vi "XVC_SERVER_UDPV3.vi"() -> ()   [LabVIEW 2017]
panel:
  out "字符串 3":string
  out "错误输出 3":errorcluster={"status"=TRUE, "code"=56, "source"="XVC_SERVER_UDPV3.vi中的读取TCP数据"} caption="错误输出"
  out "错误输出":errorcluster
  in  "address":string="192.168.10.35"
  out "x != 0?":bool=TRUE
  in  "Client Closed":string="The client VI closed the connection."
  in  "Stop":bool
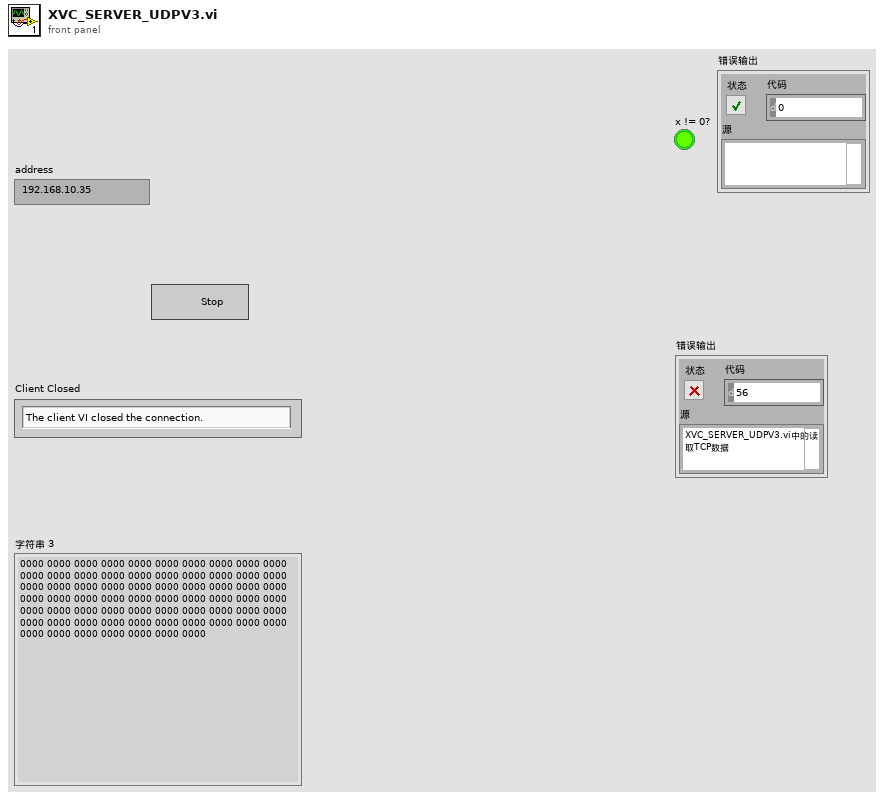
[diagram p1: front panel]
types:
  T1 = enum16{"Standard", "Buffered", "CRLF", "Immediate"}
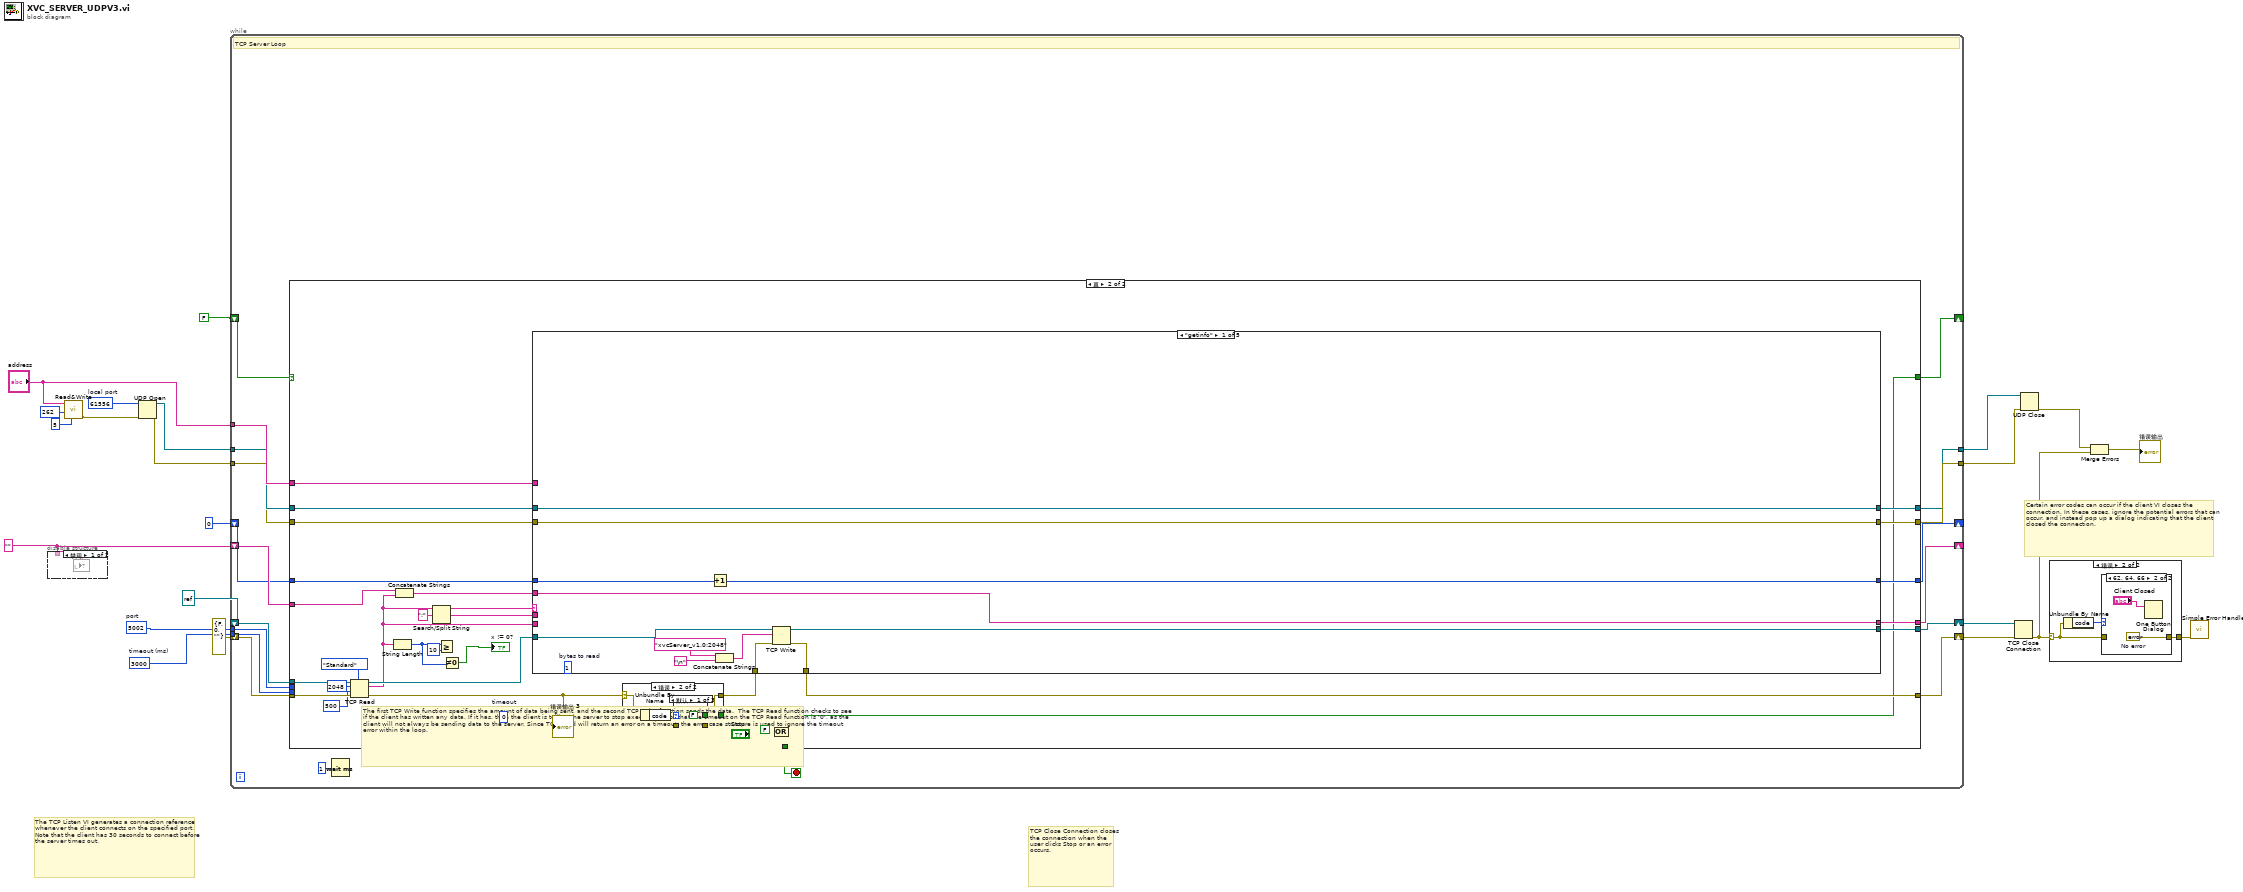
[diagram p0: block diagram]
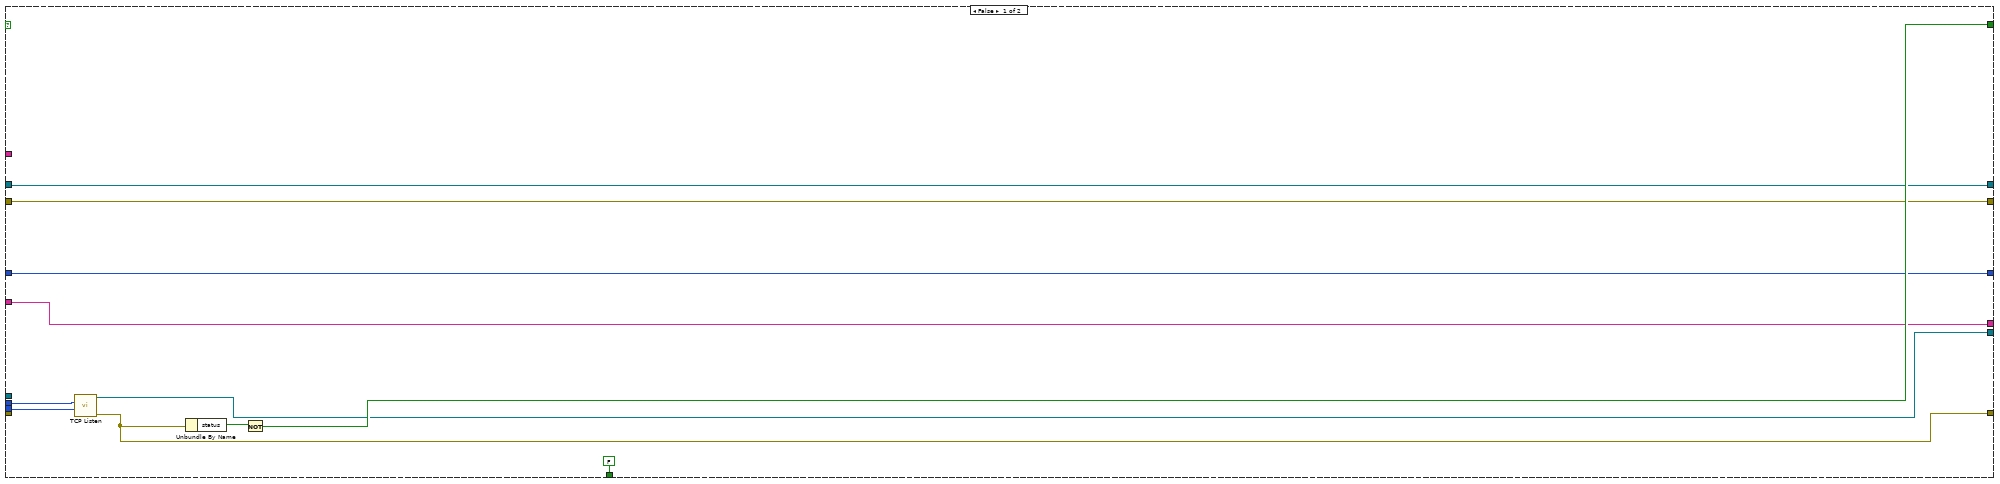
[diagram p5: hidden frame]
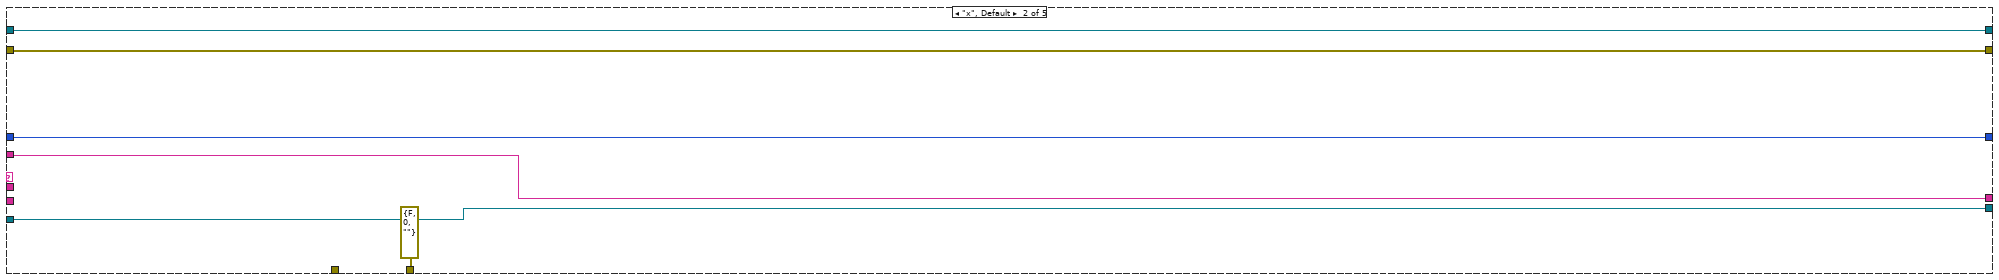
[diagram p6: hidden frame]
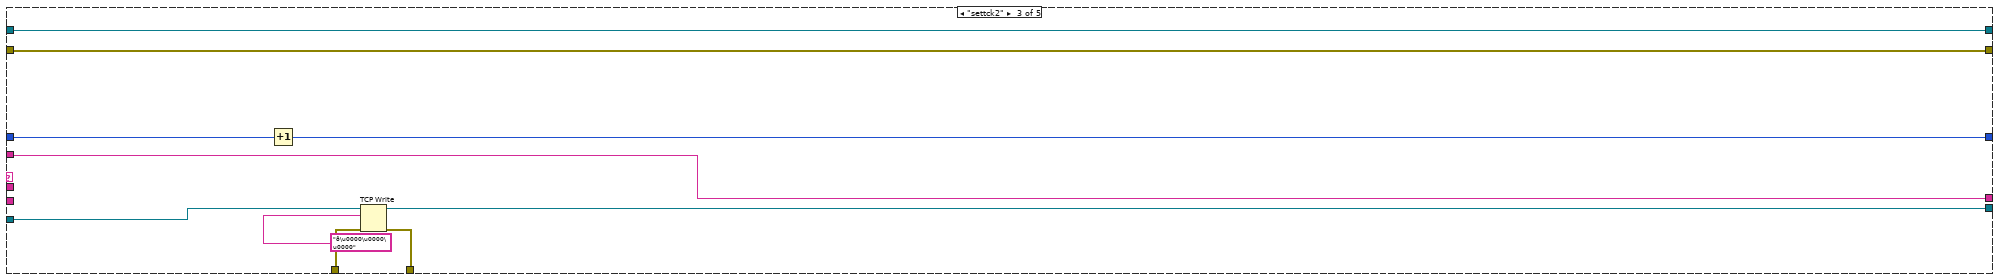
[diagram p7: hidden frame]
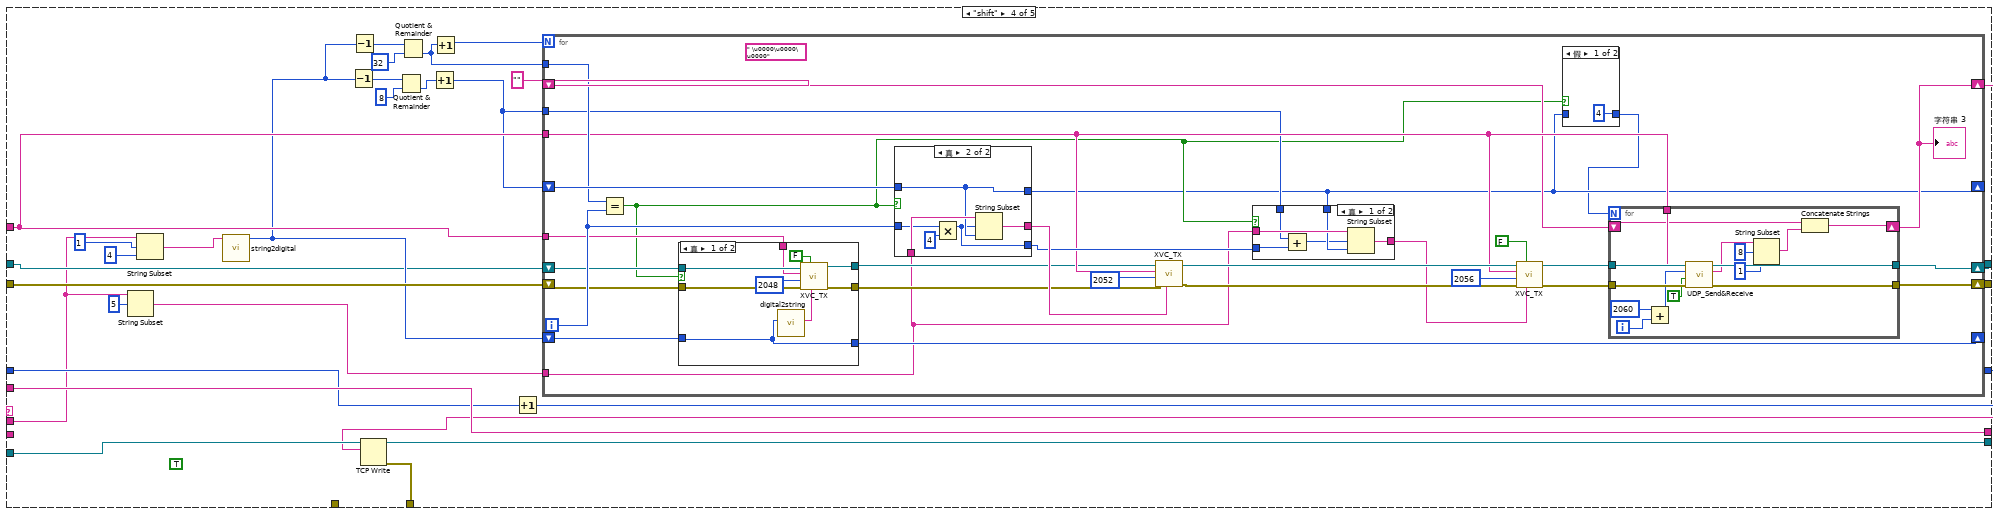
[diagram p8: hidden frame]
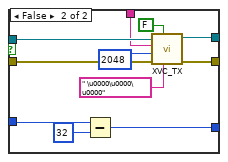
[diagram p10: hidden frame]
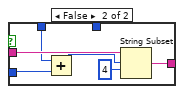
[diagram p11: hidden frame]
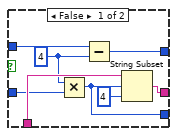
[diagram p12: hidden frame]
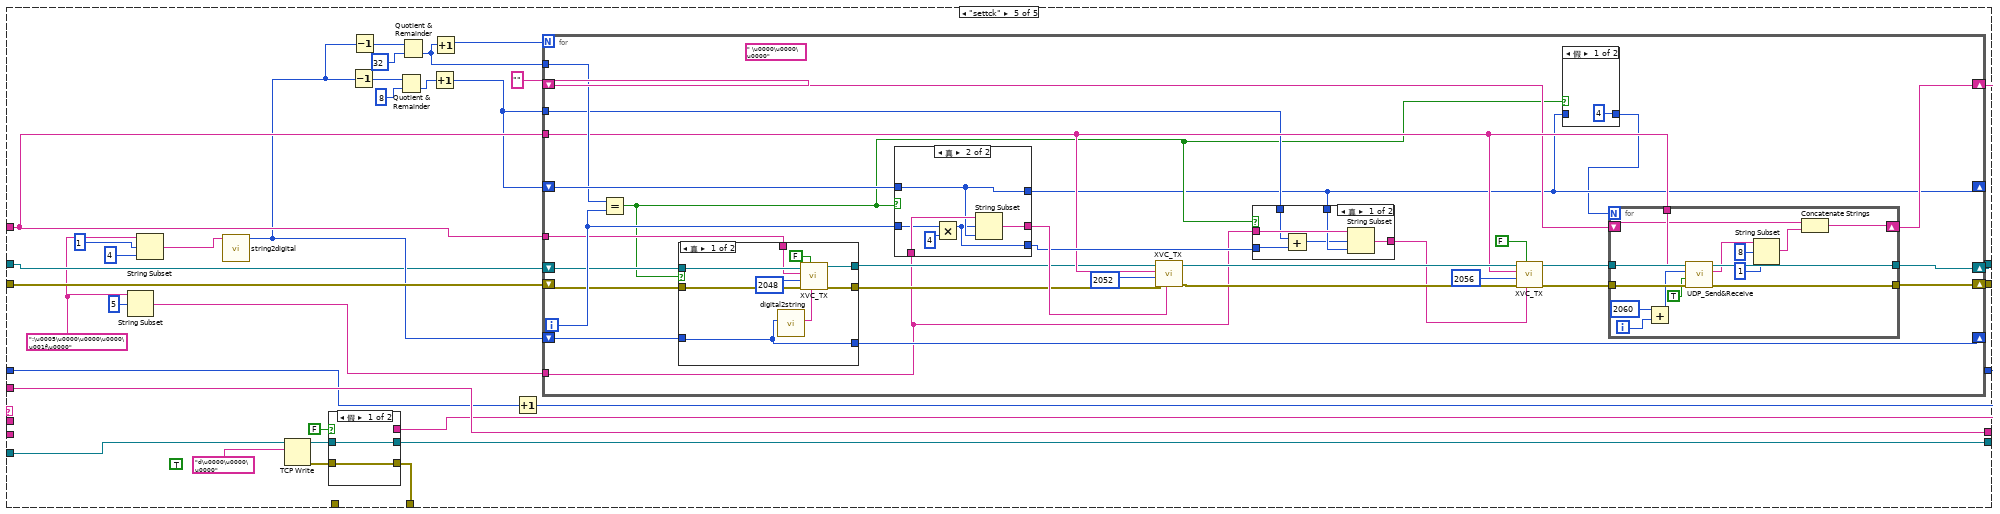
[diagram p13: hidden frame]
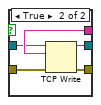
[diagram p14: hidden frame]
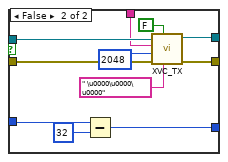
[diagram p16: hidden frame]
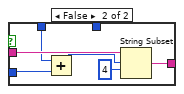
[diagram p17: hidden frame]
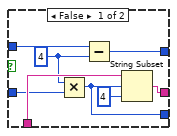
[diagram p18: hidden frame]
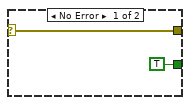
[diagram p19: hidden frame]
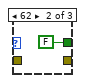
[diagram p20: hidden frame]
diagram:
  w21 = u16 61556  # local port
  w17 = ""
  w8 = u16 5002  # port
  w9 = 3000  # timeout (ms)
  # "TCP Close Connection closes the connection when the user clicks Stop or an error occurs."
  # "The TCP Listen VI generates a connection reference whenever the client connects on the specified port. Note that the client has 30 seconds to connect before the server times out."
  # "Certain error codes can occur if the client VI closes the connection. In these cases, ignore the potential errors that can occur, and instead pop up a dialog indicating that the client closed the connection."
  # "The first TCP Write function specifies the amount of data being sent, and the second TCP Write function sends the data.  The TCP Read function checks to see if the client has written any data. If it has, then the client is telling the server to stop executing. Note that the timeout on the TCP Read function is '0', as the client will not always be sending data to the server. Since TCP Read will return an error on a timeout, the error case structure is used to ignore the timeout error within the loop."
  n1 = disable-structure shown="禁用" {
    disable-tunnel: w17 -> [w23 _]
    frame Disabled {
      n2 = local write item#-1(w23) -> ()
    }
    frame Enabled {
    }
  }
  n3 = call "Read&Write.vi"("In"=u8 5, "Address"=u32 262, "address"="address") -> ("error out"=w18:errorcluster)  [unwired: 7 in, 1 out]
  n4 = UDP Open(8:w18, 11:w21) -> (port=w14:refnum<k16>, 0:w13:errorcluster)  [unwired: 3 in, 1 out]
  n5 = while {
    shift-right: [w38] -> _
    shift-left: w17 -> [w39]
    shift-right: [w36] -> _
    shift-left: u32 0 -> [w37]
    tunnel: "address" -> [w35]
    tunnel: w14 -> [w34]
    tunnel: w13 -> [w33]
    tunnel: [w32] -> w12
    tunnel: [w31] -> w11
    shift-right: [w26] -> _
    shift-left: FALSE -> [w25]
    tunnel: w9 -> [w30]
    tunnel: w8 -> [w29]
    shift-right: [w28] -> w7
    shift-left: refnum<k5> refnum ("connection ID") -> [w42]
    shift-right: [w27] -> w6
    shift-left: errorcluster {"status"=FALSE, "code"=0, "source"=""} ("error out") -> [w40]
    stop <- w41 stop-if-true
    # "TCP Server Loop"
    n6 = case shown="真" w25 {
      tunnel: w42 -> [_ w84]
      tunnel: [FALSE w83] -> w41
      tunnel: w40 -> [_ w82]
      tunnel: w39 -> [w45 w77]
      tunnel: [w49 w72] -> w27
      tunnel: [w44 w70] -> w28
      tunnel: [w45 w69] -> w38
      tunnel: w37 -> [w46 w68]
      tunnel: [w46 w66] -> w36
      tunnel: w35 -> [_ w65]
      tunnel: w34 -> [w47 w64]
      tunnel: w33 -> [w48 w63]
      tunnel: [w48 w62] -> w32
      tunnel: [w47 w61] -> w31
      tunnel: w30 -> [w53 _]
      tunnel: w29 -> [w52 _]
      tunnel: [w50 w54] -> w26
      frame False {
        n7 = call <vilib>:"TCP Listen.vi"("timeout ms (wait forever: -1)"=w53, "port"=w52) -> ("error out"=w49:errorcluster, "connection ID"=w44:refnum<k5>)  [unwired: 5 in, 3 out]
        n8 = Unbundle By Name(w49) -> ("status"=w51:bool)
        n9 = Not(x=w51) -> (.not. x?=w50:bool)
      }
      frame True {
        (unwired) 0  # timeout
        (unwired) 1  # bytes to read
        n10 = TCP Read(connection ID=w84, bytes to read=2048, error in (no error)=w82, 7:T1."Standard" ("mode (standard)"), 9:500 ("timeout ms (25000)")) -> (connection ID out=w71:refnum<k5>, data out=w57:string, error out=w80:errorcluster)
        "错误输出 3" <- w80
        n11 = String Length(string=w57) -> (length=w75:i32)
        n12 = Concatenate Strings(w77, w57) -> (w60:string)
        n13 = Search/Split String(string=w57, search string/char (-)=":" ("正则表达式")) -> (substring before match=w56:string, match + rest of string=w59:string)  [unwired: 1 in, 1 out]
        n14 = Greater Or Equal?(x=w75, y=10) -> ()  [unwired: 1 out]
        n15 = Not Equal To 0?(x=w75) -> (x != 0?=→"x != 0?":bool)
        n16 = case shown="错误" w80 {
          selector: w80 -> [w367 w370]
          tunnel: [w367 w369] -> w73
          tunnel: [TRUE ("值") w368] -> w54
          frame No Error {
          }
          frame Error {
            n17 = Unbundle By Name(w370) -> ("code"=w371:i32)
            n18 = case shown="默认" w371 {
              tunnel: w370 -> [w373 _ _]
              tunnel: [w373 _ _] -> w369
              tunnel: [FALSE ("值") FALSE ("值") TRUE ("值")] -> w368
              frame Default {
              }
              frame 62 {
              }
              frame 56 {
              }
            }
          }
        }
        n19 = case shown="\"getinfo\"" w56 {
          tunnel: w71 -> [w96 w99 w112 w140 w239]
          tunnel: w73 -> [w95 _ w110 _ _]
          tunnel: [w94 errorcluster {"status"=FALSE, "code"=0, "source"=""} ("error out") w109 w139 w265] -> w72
          tunnel: [w93 w99 w108 w138 w264] -> w70
          tunnel: [w88 w98 w103 w135 w261] -> w69
          tunnel: [w92 w100 w107 w129 w255] -> w66
          tunnel: w68 -> [w91 w100 w106 w130 w256]
          tunnel: w65 -> [_ _ _ w118 w244]
          tunnel: w64 -> [w90 w102 w105 w116 w242]
          tunnel: w63 -> [w89 w101 w104 w119 w245]
          tunnel: [w89 w101 w104 w131 w257] -> w62
          tunnel: [w90 w102 w105 w132 w258] -> w61
          tunnel: w60 -> [w88 w98 w103 w135 w261]
          tunnel: w59 -> [_ _ _ w114 _]
          tunnel: w57 -> [_ _ _ _ _]
          frame "getinfo" {
            n20 = Increment(x=w91) -> (x+1=w92:u32)
            n21 = Concatenate Strings("xvcServer_v1.0:2048", "\n") -> (w85:string)
            n22 = TCP Write(connection ID=w96, data in=w85, error in (no error)=w95) -> (connection ID out=w93:refnum<k5>, error out=w94:errorcluster)  [unwired: 1 in, 1 out]
          }
          frame "x", Default {
          }
          frame "settck2" {
            n23 = Increment(x=w106) -> (x+1=w107:u32)
            n24 = TCP Write(connection ID=w112, data in="ð\u0000\u0000\u0000", error in (no error)=w110) -> (connection ID out=w108:refnum<k5>, error out=w109:errorcluster)  [unwired: 1 in, 1 out]
          }
          frame "shift" {
            (unwired) TRUE
            n25 = String Subset(string=w114, offset (0)=5 ("偏移量(0)")) -> (substring=w123:string)  [unwired: 1 in]
            n26 = String Subset(string=w114, offset (0)=1 ("length (rest)"), length (rest)=4 ("length (rest)")) -> (substring=w133:string)
            n27 = call "string2digital.vi"("data in"=w133) -> ("number"=w117:u32)  [unwired: 10 in]
            n28 = Decrement(x=w117) -> (x-1=w124:u32)
            n29 = Decrement(x=w117) -> (x-1=w128:u32)
            n30 = Quotient & Remainder(x=w124, y=u32 8) -> (floor(x/y)=w120:u32)  [unwired: 1 out]
            n31 = Quotient & Remainder(x=w128, y=u32 32) -> (floor(x/y)=w121:u32)  [unwired: 1 out]
            n32 = Increment(x=w120) -> (x+1=w115:u32)
            n33 = Increment(x=w121) -> (x+1=w126:u32)
            n34 = Increment(x=w130) -> (x+1=w129:u32)
            n35 = for {
              N: w126 -> [_]
              tunnel: w118 -> [w155]
              shift-right: [w142] -> _
              shift-left: w115 -> [w165]
              shift-right: [w157] -> w132
              shift-left: w116 -> [w148]
              shift-right: [w156] -> w131
              shift-left: w119 -> [w152]
              tunnel: w121 -> [w164]
              tunnel: w123 -> [w144]
              shift-right: [w153] -> w113
              shift-left: "" -> [w154]
              tunnel: w118 -> [w151]
              shift-right: [w149] -> _
              shift-left: w117 -> [w150]
              tunnel: w115 -> [w145]
              i -> [w163]
              (unwired) " \u0000\u0000\u0000" ("字符串 6")
              n36 = Equal?(x=w164, y=w163) -> (x = y?=w143:bool)
              n37 = case shown="真" w143 {
                tunnel: w148 -> [w179 w190]
                tunnel: w152 -> [w178 w189]
                tunnel: w151 -> [w177 w188]
                tunnel: w150 -> [w174 w186]
                tunnel: [w174 w184] -> w149
                tunnel: [w175 w183] -> w147
                tunnel: [w173 w182] -> w146
                frame True {
                  n38 = call "digital2string.vi"("数值"=w174) -> ("字符串"=w176:string)  [unwired: 10 in]
                  n39 = call "XVC_TX.vi"("data in"=w176, "Read (TRUE)"=FALSE, "error in"=w178, "Address"=u32 2048, "IP address"=w177, "connection ID"=w179) -> ("error out"=w173:errorcluster, "connection ID 2"=w175:refnum<k16>)  [unwired: 3 in, 1 out]
                }
                frame False {
                  n40 = Subtract(x=w186, y=u32 32) -> (x-y=w184:u32)
                  n41 = call "XVC_TX.vi"("data in"=" \u0000\u0000\u0000" ("字符串 6"), "Read (TRUE)"=FALSE, "error in"=w189, "Address"=u32 2048, "IP address"=w188, "connection ID"=w190) -> ("error out"=w182:errorcluster, "connection ID 2"=w183:refnum<k16>)  [unwired: 3 in, 1 out]
                }
              }
              n42 = case shown="真" w143 {
                tunnel: w165 -> [w227 w232]
                tunnel: [w226 w232] -> w142
                tunnel: w144 -> [w225 w233]
                tunnel: w163 -> [w223 w231]
                tunnel: [w222 w229] -> w162
                tunnel: [w221 w228] -> w160
                frame False {
                  w224 = u32 4 ("y")
                  n43 = Multiply(x=w224, y=w223) -> (x*y=w221:u32)
                  n44 = Subtract(x=w227, y=w224) -> (x-y=w226:u32)
                  n45 = String Subset(string=w225, offset (0)=w221, length (rest)=4 ("长度（剩余）")) -> (substring=w222:string)
                }
                frame True {
                  n46 = Multiply(x=w231, y=4) -> (x*y=w228:i32)
                  n47 = String Subset(string=w233, offset (0)=w228, length (rest)=w232) -> (substring=w229:string)
                }
              }
              n48 = call "XVC_TX.vi"("data in"=w162, "error in"=w146, "Address"=u32 2052, "IP address"=w155, "connection ID"=w147) -> ("error out"=w166:errorcluster, "connection ID 2"=w167:refnum<k16>)  [unwired: 4 in, 1 out]
              n49 = case shown="真" w143 {
                tunnel: w144 -> [w213 w219]
                tunnel: [w212 w217] -> w161
                tunnel: w160 -> [w211 w216]
                tunnel: w142 -> [w210 _]
                tunnel: w145 -> [w209 w214]
                frame True {
                  n50 = Add(x=w209, y=w211) -> (x+y=w208:u32)
                  n51 = String Subset(string=w213, offset (0)=w208, length (rest)=w210) -> (substring=w212:string)
                }
                frame False {
                  n52 = Add(x=w214, y=w216) -> (x+y=w215:u32)
                  n53 = String Subset(string=w219, offset (0)=w215, length (rest)=4 ("长度（剩余）")) -> (substring=w217:string)
                }
              }
              n54 = call "XVC_TX.vi"("data in"=w161, "Read (TRUE)"=FALSE, "error in"=w166, "Address"=u32 2056, "IP address"=w155, "connection ID"=w167) -> ("error out"=w158:errorcluster, "connection ID 2"=w159:refnum<k16>)  [unwired: 3 in, 1 out]
              n55 = case shown="假" w143 {
                tunnel: w142 -> [_ w172]
                tunnel: [u32 4 w172] -> w141
                frame False {
                }
                frame True {
                }
              }
              n56 = for {
                N: w141 -> [_]
                tunnel: w159 -> [w207]
                tunnel: w158 -> [w206]
                tunnel: w155 -> [w205]
                shift-right: [w200] -> w153
                shift-left: w154 -> [w193]
                tunnel: [w199] -> w156
                tunnel: [w198] -> w157
                i -> [w201]
                n57 = Add(x=u32 2060 ("Address"), y=w201) -> (x+y=w202:u32)
                n58 = call "UDP_Send&Receive.vi"("connection ID"=w207, "error in (no error)"=w206, "Read (TRUE)"=TRUE, "Address"=w202, "IP address"=w205) -> ("error out"=w199:errorcluster, "received string"=w197:string, "connection ID out"=w198:refnum<k16>)  [unwired: 2 in, 1 out]
                n59 = String Subset(string=w197, offset (0)=8 ("偏移量(0)"), length (rest)=1 ("长度（剩余）")) -> (substring=w194:string)
                n60 = Concatenate Strings(w193, w194) -> (w200:string)
              }
              "字符串 3" <- w153
            }
            n61 = TCP Write(connection ID=w140, data in=w113) -> (connection ID out=w138:refnum<k5>, error out=w139:errorcluster)  [unwired: 2 in, 1 out]
          }
          frame "settck" {
            w236 = ":\u0005\u0000\u0000\u0000\u001f\u0000" ("字符串 12")
            (unwired) TRUE
            n62 = String Subset(string=w236, offset (0)=5 ("偏移量(0)")) -> (substring=w249:string)  [unwired: 1 in]
            n63 = String Subset(string=w236, offset (0)=1 ("length (rest)"), length (rest)=4 ("length (rest)")) -> (substring=w259:string)
            n64 = call "string2digital.vi"("data in"=w259) -> ("number"=w243:u32)  [unwired: 10 in]
            n65 = TCP Write(connection ID=w239, data in="d\u0000\u0000\u0000") -> (connection ID out=w235:refnum<k5>, error out=w237:errorcluster)  [unwired: 2 in, 1 out]
            n66 = Decrement(x=w243) -> (x-1=w250:u32)
            n67 = Decrement(x=w243) -> (x-1=w254:u32)
            n68 = Quotient & Remainder(x=w250, y=u32 8) -> (floor(x/y)=w246:u32)  [unwired: 1 out]
            n69 = Quotient & Remainder(x=w254, y=u32 32) -> (floor(x/y)=w247:u32)  [unwired: 1 out]
            n70 = Increment(x=w246) -> (x+1=w241:u32)
            n71 = Increment(x=w247) -> (x+1=w252:u32)
            n72 = Increment(x=w256) -> (x+1=w255:u32)
            n73 = for {
              N: w252 -> [_]
              tunnel: w244 -> [w287]
              shift-right: [w274] -> _
              shift-left: w241 -> [w297]
              shift-right: [w289] -> w258
              shift-left: w242 -> [w280]
              shift-right: [w288] -> w257
              shift-left: w245 -> [w284]
              tunnel: w247 -> [w296]
              tunnel: w249 -> [w276]
              shift-right: [w285] -> w240
              shift-left: "" -> [w286]
              tunnel: w244 -> [w283]
              shift-right: [w281] -> _
              shift-left: w243 -> [w282]
              tunnel: w241 -> [w277]
              i -> [w295]
              (unwired) " \u0000\u0000\u0000" ("字符串 6")
              n74 = Equal?(x=w296, y=w295) -> (x = y?=w275:bool)
              n75 = case shown="真" w275 {
                tunnel: w280 -> [w311 w322]
                tunnel: w284 -> [w310 w321]
                tunnel: w283 -> [w309 w320]
                tunnel: w282 -> [w306 w318]
                tunnel: [w306 w316] -> w281
                tunnel: [w307 w315] -> w279
                tunnel: [w305 w314] -> w278
                frame True {
                  n76 = call "digital2string.vi"("数值"=w306) -> ("字符串"=w308:string)  [unwired: 10 in]
                  n77 = call "XVC_TX.vi"("data in"=w308, "Read (TRUE)"=FALSE, "error in"=w310, "Address"=u32 2048, "IP address"=w309, "connection ID"=w311) -> ("error out"=w305:errorcluster, "connection ID 2"=w307:refnum<k16>)  [unwired: 3 in, 1 out]
                }
                frame False {
                  n78 = Subtract(x=w318, y=u32 32) -> (x-y=w316:u32)
                  n79 = call "XVC_TX.vi"("data in"=" \u0000\u0000\u0000" ("字符串 6"), "Read (TRUE)"=FALSE, "error in"=w321, "Address"=u32 2048, "IP address"=w320, "connection ID"=w322) -> ("error out"=w314:errorcluster, "connection ID 2"=w315:refnum<k16>)  [unwired: 3 in, 1 out]
                }
              }
              n80 = case shown="真" w275 {
                tunnel: w297 -> [w359 w364]
                tunnel: [w358 w364] -> w274
                tunnel: w276 -> [w357 w365]
                tunnel: w295 -> [w355 w363]
                tunnel: [w354 w361] -> w294
                tunnel: [w353 w360] -> w292
                frame False {
                  w356 = u32 4 ("y")
                  n81 = Multiply(x=w356, y=w355) -> (x*y=w353:u32)
                  n82 = Subtract(x=w359, y=w356) -> (x-y=w358:u32)
                  n83 = String Subset(string=w357, offset (0)=w353, length (rest)=4 ("长度（剩余）")) -> (substring=w354:string)
                }
                frame True {
                  n84 = Multiply(x=w363, y=4) -> (x*y=w360:i32)
                  n85 = String Subset(string=w365, offset (0)=w360, length (rest)=w364) -> (substring=w361:string)
                }
              }
              n86 = call "XVC_TX.vi"("data in"=w294, "error in"=w278, "Address"=u32 2052, "IP address"=w287, "connection ID"=w279) -> ("error out"=w298:errorcluster, "connection ID 2"=w299:refnum<k16>)  [unwired: 4 in, 1 out]
              n87 = case shown="真" w275 {
                tunnel: w276 -> [w345 w351]
                tunnel: [w344 w349] -> w293
                tunnel: w292 -> [w343 w348]
                tunnel: w274 -> [w342 _]
                tunnel: w277 -> [w341 w346]
                frame True {
                  n88 = Add(x=w341, y=w343) -> (x+y=w340:u32)
                  n89 = String Subset(string=w345, offset (0)=w340, length (rest)=w342) -> (substring=w344:string)
                }
                frame False {
                  n90 = Add(x=w346, y=w348) -> (x+y=w347:u32)
                  n91 = String Subset(string=w351, offset (0)=w347, length (rest)=4 ("长度（剩余）")) -> (substring=w349:string)
                }
              }
              n92 = call "XVC_TX.vi"("data in"=w293, "Read (TRUE)"=FALSE, "error in"=w298, "Address"=u32 2056, "IP address"=w287, "connection ID"=w299) -> ("error out"=w290:errorcluster, "connection ID 2"=w291:refnum<k16>)  [unwired: 3 in, 1 out]
              n93 = case shown="假" w275 {
                tunnel: w274 -> [_ w304]
                tunnel: [u32 4 w304] -> w273
                frame False {
                }
                frame True {
                }
              }
              n94 = for {
                N: w273 -> [_]
                tunnel: w291 -> [w339]
                tunnel: w290 -> [w338]
                tunnel: w287 -> [w337]
                shift-right: [w332] -> w285
                shift-left: w286 -> [w325]
                tunnel: [w331] -> w288
                tunnel: [w330] -> w289
                i -> [w333]
                n95 = Add(x=u32 2060 ("Address"), y=w333) -> (x+y=w334:u32)
                n96 = call "UDP_Send&Receive.vi"("connection ID"=w339, "error in (no error)"=w338, "Read (TRUE)"=TRUE, "Address"=w334, "IP address"=w337) -> ("error out"=w331:errorcluster, "received string"=w329:string, "connection ID out"=w330:refnum<k16>)  [unwired: 2 in, 1 out]
                n97 = String Subset(string=w329, offset (0)=8 ("偏移量(0)"), length (rest)=1 ("长度（剩余）")) -> (substring=w326:string)
                n98 = Concatenate Strings(w325, w326) -> (w332:string)
              }
            }
            n99 = case shown="假" FALSE {
              tunnel: [w266 w272] -> w265
              tunnel: [w267 w271] -> w264
              tunnel: w240 -> [_ w270]
              tunnel: w237 -> [w266 w269]
              tunnel: w235 -> [w267 w268]
              frame False {
              }
              frame True {
                n100 = TCP Write(connection ID=w268, data in=w270, error in (no error)=w269) -> (connection ID out=w271:refnum<k5>, error out=w272:errorcluster)  [unwired: 1 in, 1 out]
              }
            }
          }
        }
        n101 = Compound Arithmetic op=OR(FALSE ("值"), "Stop") -> (w83:bool)
      }
    }
    n102 = Wait (ms)(milliseconds to wait=u32 1 ("等待时间（毫秒）")) -> ()  [unwired: 1 out]
  }
  n103 = TCP Close Connection(connection ID=w7, error in (no error)=w6) -> (error out=w2:errorcluster)  [unwired: 2 out]
  n104 = UDP Close(connection ID=w11, 8:w12) -> (error out=w3:errorcluster)  [unwired: 1 out]
  n105 = case shown="错误" w2 {
    selector: w2 -> [w376 w378]
    tunnel: [w376 w377] -> w22
    frame No Error {
    }
    frame Error {
      n106 = Unbundle By Name(w378) -> ("code"=w379:i32)
      n107 = case shown="62, 64, 66" w379 {
        tunnel: w378 -> [w380 _]
        tunnel: [w380 w382] -> w377
        frame Default {
        }
        frame 62, 64, 66 {
          w382 = errorcluster {"status"=FALSE, "code"=0, "source"=""}  # No error
          n108 = One Button Dialog(message="Client Closed") -> ()  [unwired: 1 in, 1 out]
        }
      }
    }
  }
  n109 = Merge Errors(w3, w2) -> (→"错误输出":errorcluster)
  n110 = call <vilib>:"Simple Error Handler.vi"("error in (no error)"=w22) -> ()  [unwired: 1 in, 8 out]
